vi "Parse CSV From cRIO.vi"(0 "/path/":string="/auton/", 1 "File Name":string, 4 "Header Row?":bool=TRUE) -> (5 "Output Array":dbl[][](array[numeric]))   [LabVIEW 2012]
uses:
  <vilib>/Utility/file.llb/Read From Spreadsheet File (string).vi
panel:
  out "Path and file":string
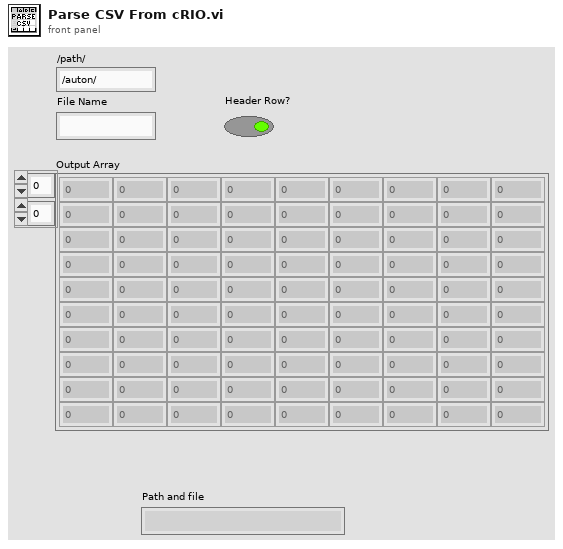
[diagram p1: front panel]
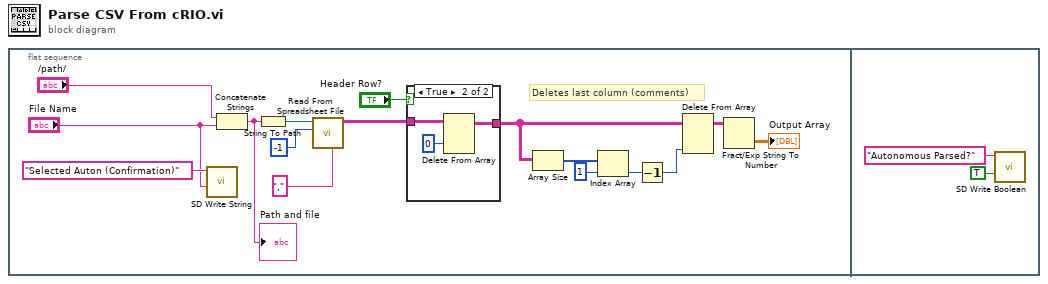
[diagram p0: block diagram]
diagram:
  n1 = flat-sequence {
    frame #0 {
      # "Deletes last column (comments)"
      n2 = call <vilib>:"SD Write String.vi"("String"="File Name", "Name"="Selected Auton (Confirmation)") -> ()  [unwired: 8 in, 2 out]
      n3 = Concatenate Strings("/path/", "File Name") -> (w13:string)
      "Path and file" <- w13
      n4 = String To Path(string=w13) -> (path=w12:path)
      n5 = call-poly <vilib>:"Read From Spreadsheet File.vi"("delimiter (\\t)"="," ("delimiter (\\t)"), "number of rows (all:-1)"=-1, "file path (dialog if empty)"=w12) -> ("all rows"=w11:string[][])  [unwired: 2 in, 6 out]
      n6 = case shown="True" "Header Row?" {
        tunnel: w11 -> [w17 w20]
        tunnel: [w17 w18] -> w5
        frame False {
        }
        frame True {
          n7 = Delete From Array(array=w20, index (row)=0) -> (array with subset deleted=w18:string[][])  [unwired: 2 in, 1 out]
        }
      }
      n8 = Array Size(array=w5) -> (size(s)=w9:i32[])
      n9 = Index Array "Index Array"(array=w9, index=1) -> (element=w7:i32)
      n10 = Decrement(x=w7) -> (x-1=w6:i32)
      n11 = Delete From Array(array=w5, index (col)=w6) -> (array with subset deleted=w4:string[][])  [unwired: 2 in, 1 out]
      n12 = Fract/Exp String To Number(string=w4) -> (number=→"Output Array":dbl[][])  [unwired: 3 in, 1 out]
    }
    frame #1 {
      n13 = call <vilib>:"SD Write Boolean.vi"("Boolean"=TRUE, "Name"="Autonomous Parsed?") -> ()  [unwired: 8 in, 2 out]
    }
  }
